vi "GEN_Load Fail Clue Info.vi"(8 "error in (no error)":errorcluster caption="错误输入（无错误）", 11 "Failed LoadedT":cluster{"Thread Name":string, "Fail?":bool}[](array[cluster])) -> (0 "error out":errorcluster caption="错误输出", 2 "User Clue out":string)   [LabVIEW 2016]
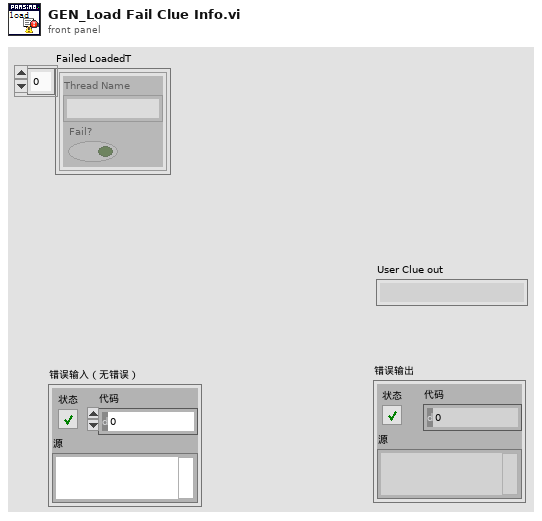
[diagram p1: front panel]
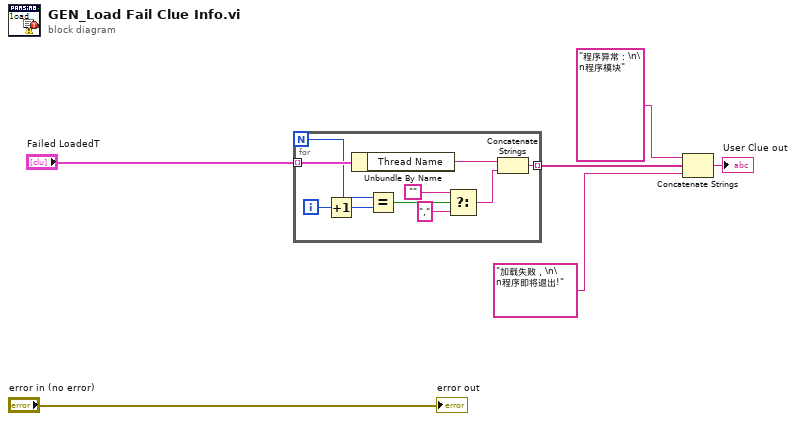
[diagram p0: block diagram]
diagram:
  n1 = for {
    N -> [w12]
    tunnel: "Failed LoadedT" -> [w16] mode=indexing
    tunnel: [w7] -> w5 mode=indexing
    i -> [w14]
    n2 = Increment(x=w14) -> (x+1=w13:i32)
    n3 = Unbundle By Name(w16) -> ("Thread Name"=w15:string)
    n4 = Equal?(x=w12, y=w13) -> (x = y?=w11:bool)
    n5 = Select(t="", s=w11, f=",") -> (s? t:f=w8:string)
    n6 = Concatenate Strings(w15, w8) -> (w7:string)
  }
  n7 = Concatenate Strings("程序异常：\n\n程序模块" ("f"), w5, "加载失败，\n\n程序即将退出!" ("f")) -> (→"User Clue out":string)
  "error out" <- "error in (no error)"
